vi "Pressurized Reaction Chamber.vi"(7 "Speed Upgrades":u32 max=8, 9 "In Gas (mB/t)":u32, 10 "Water (mB/t)":u32, 11 "Input":u16(ring) items=["Coal", "Coal Block", "Pu/Po"]) -> (0 "Limiting":bool, 1 "B Limiting":bool, 2 "A Limiting":bool, 3 "Produced Items/t":ext, 4 "Required Items/t":ext, 5 "Out Gas (mB/t)":u32, 6 "Required Items/s":ext)   [LabVIEW 2023]
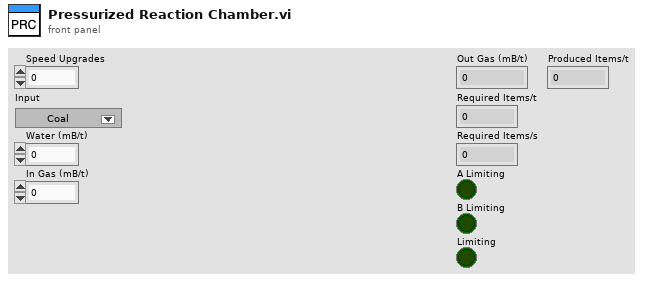
[diagram p1: front panel]
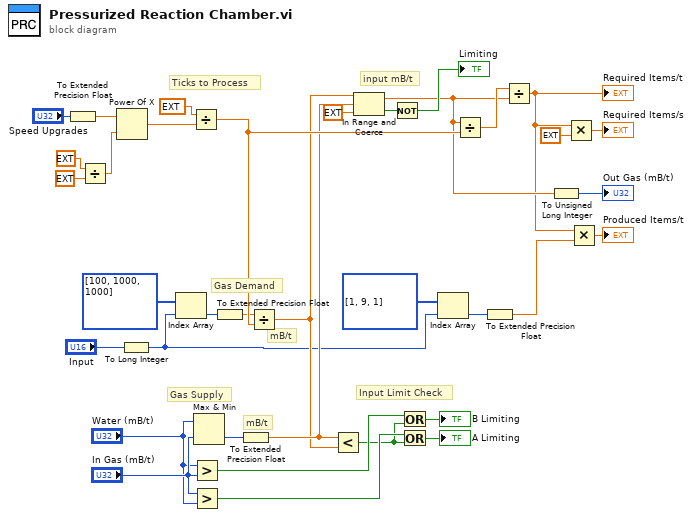
[diagram p0: block diagram]
diagram:
  # "input mB/t"
  # "mB/t"
  # "mB/t"
  # "Input Limit Check"
  # "Gas Supply"
  # "Gas Demand"
  # "Ticks to Process"
  n1 = To Extended Precision Float(1:"Speed Upgrades") -> (0:w28:ext)
  n2 = Divide(x=ext 4.0, y=ext 3.0) -> (x/y=w31:ext)
  n3 = Power Of X(1:w31, 2:w28) -> (0:w35:ext)
  n4 = To Long Integer(number="Input") -> (32bit integer=w5:i32)
  n5 = Index Array(array=u32[] [100, 1000, 1000], index=w5) -> (element=w14:u32)
  n6 = Divide(x=ext 100.0 ("y"), y=w35) -> (x/y=w13:ext)
  n7 = Greater?(x="Water (mB/t)", y="In Gas (mB/t)") -> (0:w23:bool)
  n8 = Greater?(x="In Gas (mB/t)", y="Water (mB/t)") -> (0:w22:bool)
  n9 = Max & Min(x="Water (mB/t)", y="In Gas (mB/t)") -> (min(x,y)=w17:u32)  [unwired: 1 out]
  n10 = To Extended Precision Float(1:w14) -> (0:w12:ext)
  n11 = To Extended Precision Float(1:w17) -> (0:w11:ext)
  n12 = Divide(x=w12, y=w13) -> (x/y=w10:ext)
  n13 = Less?(x=w11, y=w10) -> (x < y?=w19:bool)
  n14 = In Range and Coerce(upper limit=w10, x=w11, lower limit=ext 0.0) -> (coerced(x)=w8:ext, In Range?=w16:bool)
  n15 = Not(x=w16) -> (.not. x?=→"Limiting":bool)
  n16 = Or(x=w23, y=w19) -> (x .or. y?=→"B Limiting":bool)
  n17 = Or(x=w22, y=w19) -> (x .or. y?=→"A Limiting":bool)
  n18 = Index Array(array=u32[] [1, 9, 1], index=w5) -> (element=w4:u32)
  n19 = Divide(x=w8, y=w13) -> (x/y=w9:ext)
  n20 = To Extended Precision Float(1:w4) -> (0:w2:ext)
  n21 = Divide(x=w9, y=w8) -> (x/y=w3:ext)
  "Required Items/t" <- w3
  n22 = To Unsigned Long Integer(number=w8) -> (unsigned 32bit integer=→"Out Gas (mB/t)":u32)
  n23 = Multiply(x=w3, y=ext 20.0) -> (x*y=→"Required Items/s":ext)
  n24 = Multiply(x=w3, y=w2) -> (x*y=→"Produced Items/t":ext)
